vi "挥发酚启动命令.vi"(11 "参数":T1={"站号"=21, "量程切换"=enum."AUTO", "控制命令"=0, "模式设置"=enum."待机", "测量间隔"=0} {"站号" items=["挥发酚"=1, "总氮"=2, "氨氮"=3]; "控制命令" items=["启动测量"=1, "标样核查"=2, "零点核查"=3, "跨度核查"=4, "空白测试"=5, "平行样测试"=6, "加标回收"=7, "空白校准"=8, "标样校准"=9, "初始化（清洗）"=10, "停止测试"=11, "仪器重启"=12, "校时"=13, "模式设置"=14, "测量间隔设置"=15, "调试"=22, "填充管路"=30, "清洗管路"=31, "清洗反应杯"=32]}) -> (3 "启动命令":cluster{"命令":string, "data":variant})   [LabVIEW 2022 SP3, in "挥发酚.lvlib"]
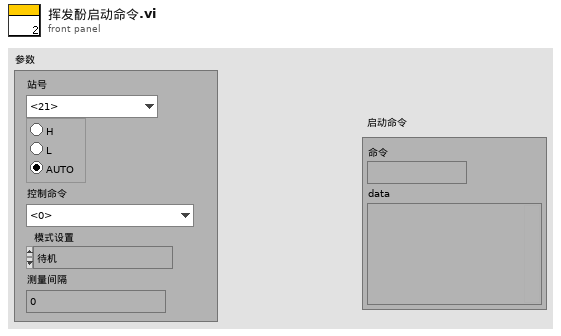
[diagram p1: front panel]
types:
  T1 = cluster{"站号":u16, "量程切换":enum32{"H", "L", "AUTO"}, "控制命令":u16, "模式设置":enum16{"待机", "连续模式", "周期模式", "定点模式", "受控模式", "手动模式"}, "测量间隔":u16}
  T2 = enum16{"待机", "连续模式", "周期模式", "定点模式", "受控模式", "手动模式"}
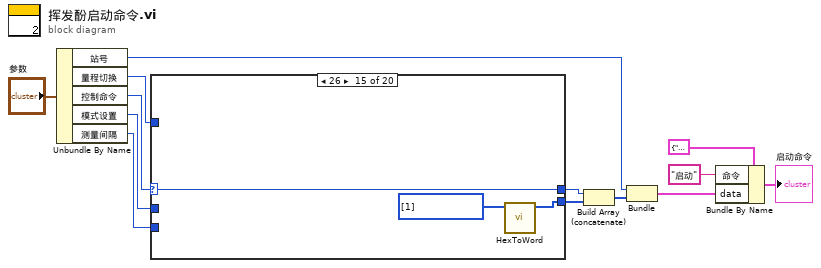
[diagram p0: block diagram]
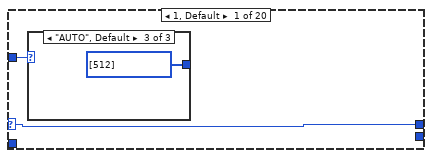
[diagram p2: hidden frame]
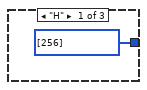
[diagram p3: hidden frame]
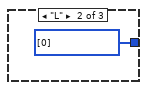
[diagram p4: hidden frame]
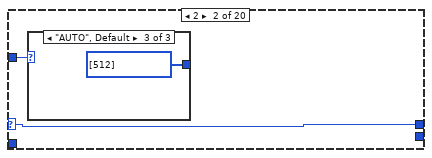
[diagram p5: hidden frame]
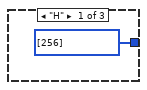
[diagram p6: hidden frame]
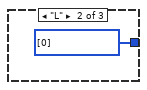
[diagram p7: hidden frame]
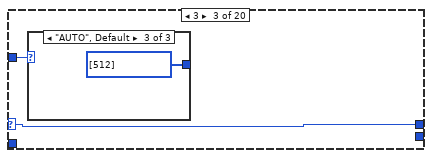
[diagram p8: hidden frame]
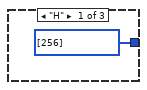
[diagram p9: hidden frame]
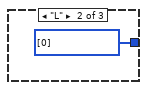
[diagram p10: hidden frame]
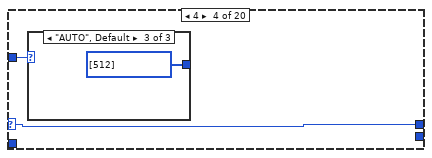
[diagram p11: hidden frame]
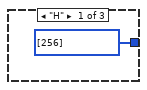
[diagram p12: hidden frame]
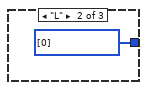
[diagram p13: hidden frame]
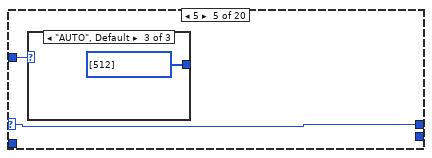
[diagram p14: hidden frame]
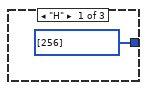
[diagram p15: hidden frame]
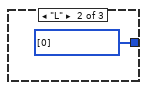
[diagram p16: hidden frame]
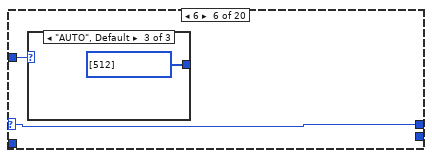
[diagram p17: hidden frame]
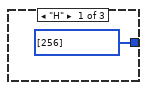
[diagram p18: hidden frame]
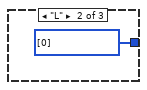
[diagram p19: hidden frame]
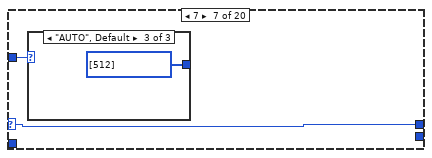
[diagram p20: hidden frame]
diagram:
  n1 = Unbundle By Name("参数") -> ("站号"=w11:u16, "量程切换"=w10:enum32{"H", "L", "AUTO"}, "控制命令"=w9:u16, "模式设置"=w7:T2, "测量间隔"=w8:u16)
  n2 = case shown="26" w9 {
    selector: w9 -> [w14 w19 w24 w29 w34 w39 w44 w49 w54 w59 w60 w61 w63 w69 w78 w80 w85 w90 w95 w100]
    tunnel: w10 -> [w15 w20 w25 w30 w35 w40 w45 w50 w55 _ _ _ _ _ _ _ w84 _ _ _]
    tunnel: [w14 w19 w24 w29 w34 w39 w44 w49 w54 w59 w60 w61 w63 w69 w78 w80 w85 w90 w95 w100] -> w3
    tunnel: w8 -> [_ _ _ _ _ _ _ _ _ _ _ _ _ _ _ w81 _ _ _ _]
    tunnel: w7 -> [_ _ _ _ _ _ _ _ _ _ _ _ _ _ _ _ _ _ _ _]
    tunnel: [_ _ _ _ _ _ _ _ _ _ _ _ w62 w67 w77 _ _ _ _ _] -> w1
    frame 1, Default {
      n3 = case shown="\"AUTO\", Default" w15 {
        tunnel: [i32[] [256] i32[] [0] i32[] [512]] -> _
        frame "H" {
        }
        frame "L" {
        }
        frame "AUTO", Default {
        }
      }
    }
    frame 2 {
      n4 = case shown="\"AUTO\", Default" w20 {
        tunnel: [i32[] [256] i32[] [0] i32[] [512]] -> _
        frame "H" {
        }
        frame "L" {
        }
        frame "AUTO", Default {
        }
      }
    }
    frame 3 {
      n5 = case shown="\"AUTO\", Default" w25 {
        tunnel: [i32[] [256] i32[] [0] i32[] [512]] -> _
        frame "H" {
        }
        frame "L" {
        }
        frame "AUTO", Default {
        }
      }
    }
    frame 4 {
      n6 = case shown="\"AUTO\", Default" w30 {
        tunnel: [i32[] [256] i32[] [0] i32[] [512]] -> _
        frame "H" {
        }
        frame "L" {
        }
        frame "AUTO", Default {
        }
      }
    }
    frame 5 {
      n7 = case shown="\"AUTO\", Default" w35 {
        tunnel: [i32[] [256] i32[] [0] i32[] [512]] -> _
        frame "H" {
        }
        frame "L" {
        }
        frame "AUTO", Default {
        }
      }
    }
    frame 6 {
      n8 = case shown="\"AUTO\", Default" w40 {
        tunnel: [i32[] [256] i32[] [0] i32[] [512]] -> _
        frame "H" {
        }
        frame "L" {
        }
        frame "AUTO", Default {
        }
      }
    }
    frame 7 {
      n9 = case shown="\"AUTO\", Default" w45 {
        tunnel: [i32[] [256] i32[] [0] i32[] [512]] -> _
        frame "H" {
        }
        frame "L" {
        }
        frame "AUTO", Default {
        }
      }
    }
    frame 8 {
      n10 = case shown="\"AUTO\", Default" w50 {
        tunnel: [i32[] [256] i32[] [0] i32[] [512]] -> _
        frame "H" {
        }
        frame "L" {
        }
        frame "AUTO", Default {
        }
      }
    }
    frame 9 {
      n11 = case shown="\"AUTO\", Default" w55 {
        tunnel: [i32[] [256] i32[] [0] i32[] [512]] -> _
        frame "H" {
        }
        frame "L" {
        }
        frame "AUTO", Default {
        }
      }
    }
    frame 10 {
      (unwired) i32[] []
    }
    frame 11 {
      (unwired) i32[] []
    }
    frame 12 {
      (unwired) i32[] []
    }
    frame 13 {
      n12 = Get Date/Time In Seconds() -> (seconds since 1Jan1904=w66:timestamp)
      n13 = Insert Into Array(array=timestamp[] [] ("数组"), new element=w66) -> (w64:timestamp[])  [unwired: 1 in]
      n14 = call "DateToHex.vi"("DATE"=w64) -> ("数组"=w62:u16[])  [unwired: 10 in]
    }
    frame 14 {
      n15 = case shown="\"受控模式\"" T2."受控模式" ("模式设置") {
        tunnel: [i32[] [0] i32[] [1] i32[] [2] i32[] [3] i32[] [4] i32[] [5]] -> w70
        frame "待机", Default {
        }
        frame "连续模式" {
        }
        frame "周期模式" {
        }
        frame "定点模式" {
        }
        frame "受控模式" {
        }
        frame "手动模式" {
        }
      }
      n16 = call "HexToWord.vi"("数组"=w70) -> ("WORD"=w67:u16[])  [unwired: 10 in]
    }
    frame 26 {
      n17 = call "HexToWord.vi"("数组"=i32[] [1]) -> ("WORD"=w77:u16[])  [unwired: 10 in]
    }
    frame 15 {
      n18 = Replace Array Subset(array=i32[] [0], new element=w81) -> (w82:i32[])  [unwired: 1 in]
      n19 = call "HexToWord.vi"("数组"=w82) -> ()  [unwired: 10 in, 1 out]
    }
    frame 22 {
      n20 = case shown="\"L\"" w84 {
        tunnel: [i32[] [256] i32[] [0] i32[] [512]] -> _
        frame "H" {
        }
        frame "L" {
        }
        frame "AUTO", Default {
        }
      }
    }
    frame 30 {
      n21 = case shown="\"L\"" enum32{"H", "L", "AUTO"}."L" ("量程切换") {
        tunnel: [i32[] [256] i32[] [0] i32[] [512]] -> _
        frame "H" {
        }
        frame "L" {
        }
        frame "AUTO", Default {
        }
      }
    }
    frame 31 {
      n22 = case shown="\"L\"" enum32{"H", "L", "AUTO"}."L" ("量程切换") {
        tunnel: [i32[] [256] i32[] [0] i32[] [512]] -> _
        frame "H" {
        }
        frame "L" {
        }
        frame "AUTO", Default {
        }
      }
    }
    frame 32 {
      n23 = case shown="\"L\"" enum32{"H", "L", "AUTO"}."L" ("量程切换") {
        tunnel: [i32[] [256] i32[] [0] i32[] [512]] -> _
        frame "H" {
        }
        frame "L" {
        }
        frame "AUTO", Default {
        }
      }
    }
  }
  n24 = Build Array (concatenate)(w3, w1) -> (w2:u16[])
  n25 = Bundle("站号"=w11, w2) -> (w4:cluster{"站号":u16, u16[]})  [unwired: 1 in]
  n26 = Bundle By Name(cluster=cluster{"命令":string, "data":variant} {"命令"="", "data"=variant} ("元素"), "命令"="启动", "data"=w4) -> (→"启动命令":cluster{"命令":string, "data":variant})
